vi "motion_generate_test_withvelocitycontrol_withswingdelay.vi"() -> ()   [LabVIEW 2017]
uses:
  d2619827-b21f-489f-b2a3-d550c82ff8e2.vi
  Downloads/Interfacing File 1/Software_Driver/DynamixelSDK/DynamixelSDK-master/labview/dxl_x86_c.lvlib/dxl_x86_c.lvlib
panel:
  in  "millisecond timer value":u32=200
  in  "ADDR_MX_GOAL_Velocity 2":u8=5
  in  "data 4":u16
  in  "data 3":u16
  in  "data 2":u16
  in  "data":u16
  in  "ADDR_MX_GOAL_Velocity":u8=5
  in  "angle 2":dbl=180.0
  in  "swing 2":dbl=185.0
  in  "motor3 2":dbl=220.0
  in  "motor1&2 2":dbl=150.0
  in  "z축 선택":dbl
  in  "motor1&2":dbl=150.0
  in  "motor3":dbl=220.0
  in  "swing":dbl=185.0
  in  "angle":dbl=180.0
  in  "Boolean":bool
  in  "positioning time_2":u32
  in  "positioning time_1":u32
  in  "initial_5":dbl=230.0
  in  "initial_4":dbl=180.0
  out "value : MX (knob)\npresent position 5":u16(knob)
  out "value : MX (knob)\npresent position 4":u16(knob)
  in  "dynamixel_id 5":u8=5
  in  "dynamixel_id 4":u8=4
  out "protocol_version 2":dbl=2.0
  in  "ADDR_MX_\nPRESENT_POSITION 2":u16=132
  out "dynamixel_error 2":string
  out "dynamixel_comm_result  2":string
  in  "ADDR_MX_\nGOAL_POSITION 2":u16=116
  in  "ADDR_MX_\nTORQUE_ENABLE 2":u16=64
  in  "initial_3":dbl=260.0
  in  "initial_1&2":dbl=230.0
  out "value : MX (knob)\npresent position 3":u16(knob)
  out "value : MX (knob)\npresent position 2":u16(knob)
  out "value : MX (knob)\npresent position":u16(knob)
  in  "dynamixel_id 3":u8=3
  in  "dynamixel_id 2":u8=2
  out "dynamixel_comm_result":string
  out "dynamixel_error":string
  in  "device_name":string="COM3"
  in  "ADDR_MX_\nPRESENT_POSITION":u16=36
  in  "ADDR_MX_\nGOAL_POSITION":u16=30
  in  "ADDR_MX_\nTORQUE_ENABLE":u16=24
  out "protocol_version":dbl=1.0
  in  "terminate":bool
  out "port_num":i32
  in  "dynamixel_id":u8=1
  in  "baud_rate":i32=57600
  # "Motor connection status"
  # "Time set"
  # "Sensing data"
  # "Handler setup"
  # "link length"
  # "initial angle"
  # "desired angle"
  # "*각 관절에 모터 연결 시 180도 라인 기준으로 연결 시키기 \n(-각도 반영해주기 위함!) \n-> 모터 input은 -180~180까지 계산됨!"
  # "*yaw motor는 0도 라인 기준으로 연결 시키기"
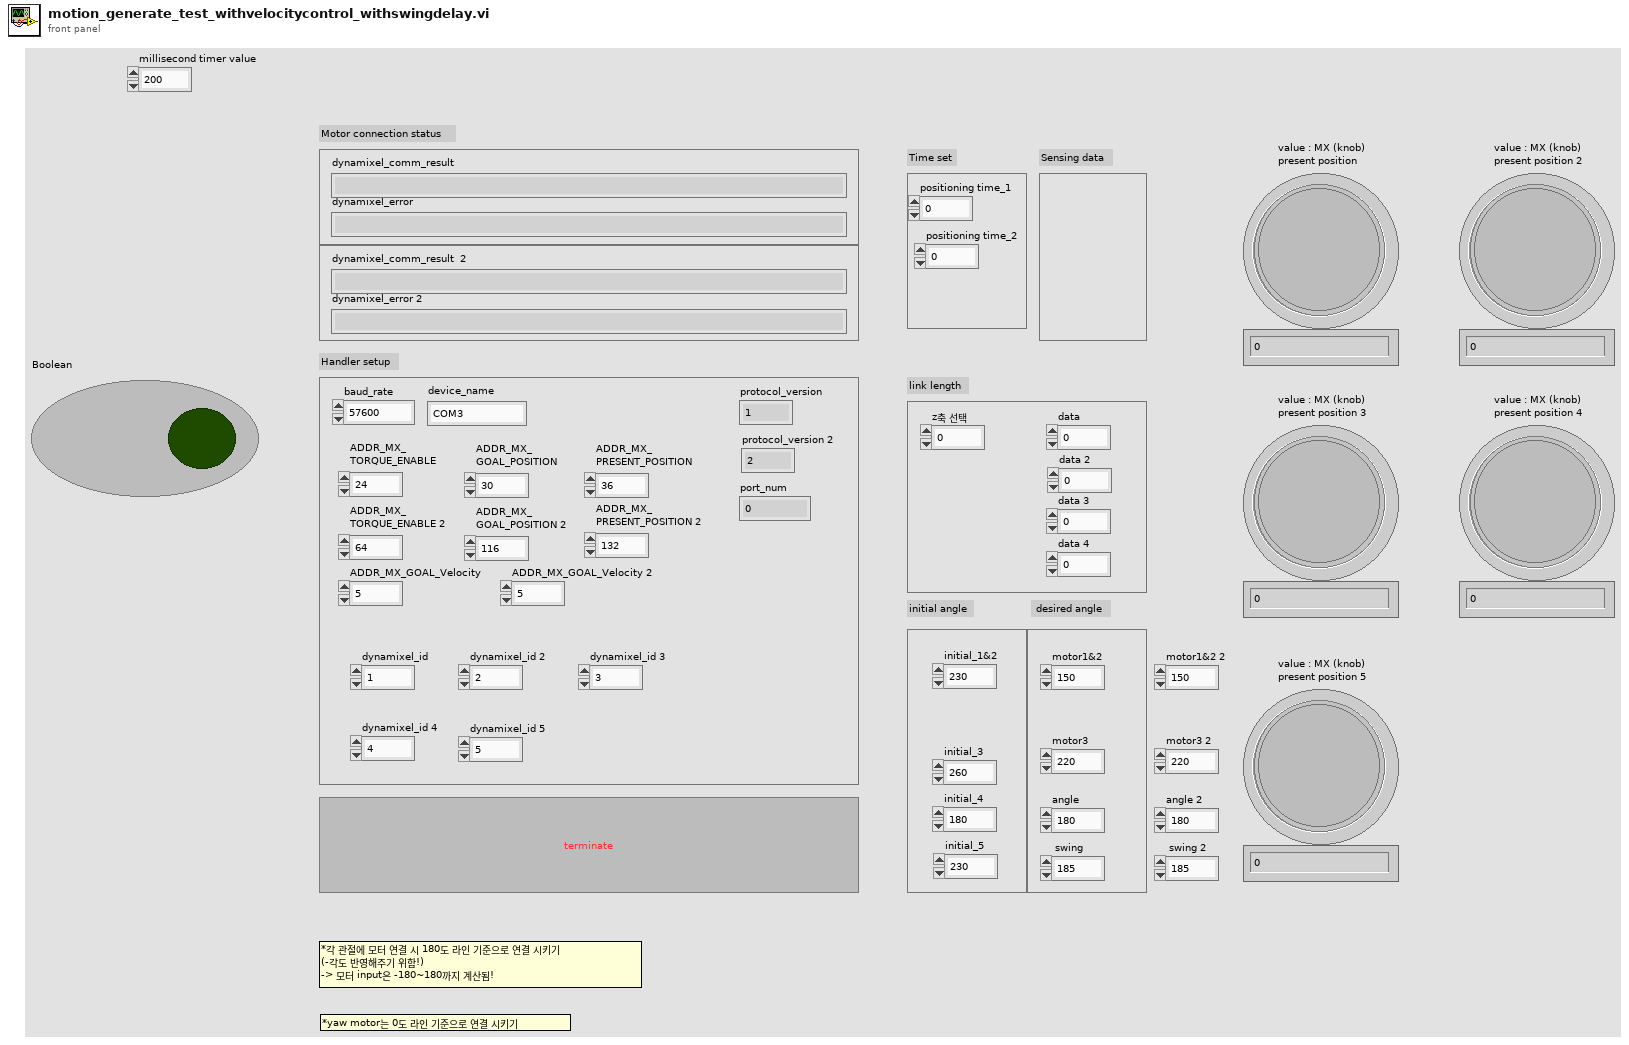
[diagram p1: front panel]
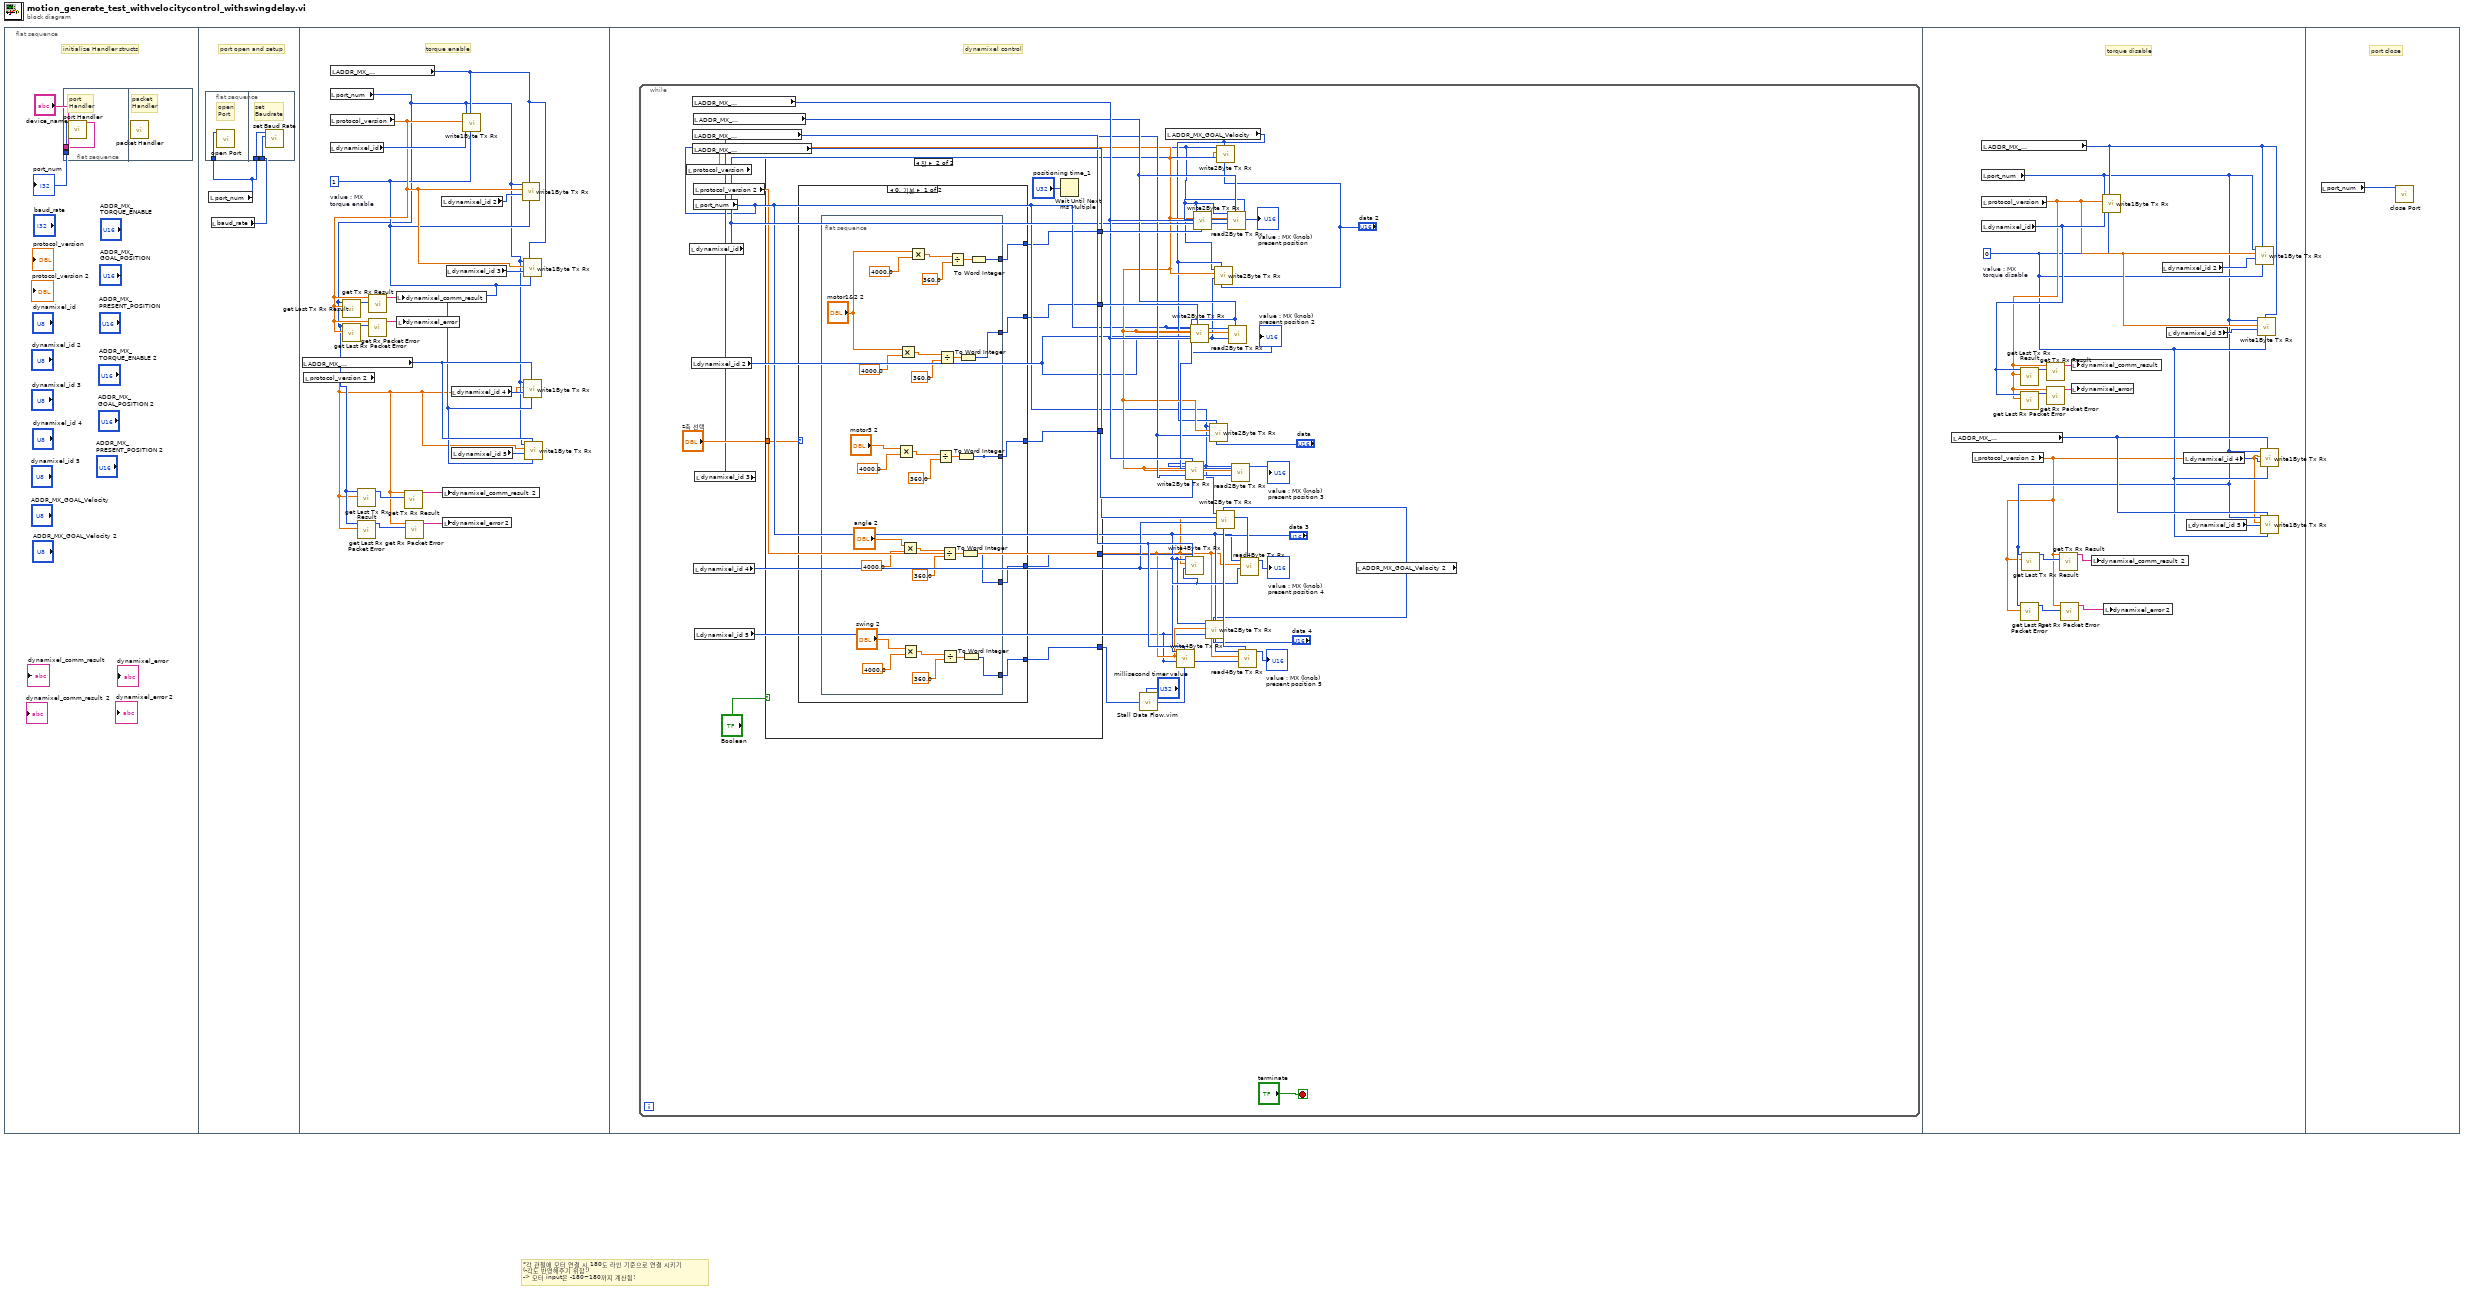
[diagram p0: block diagram]
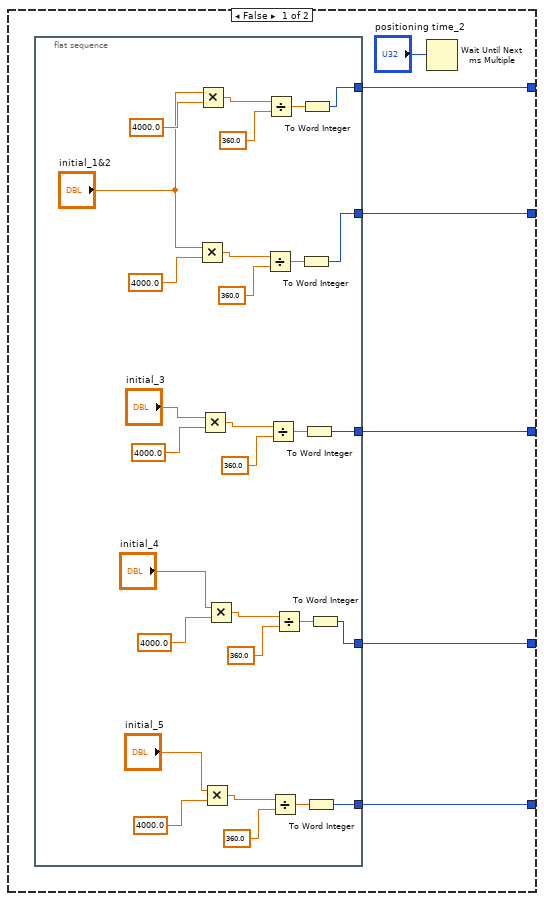
[diagram p2: hidden frame]
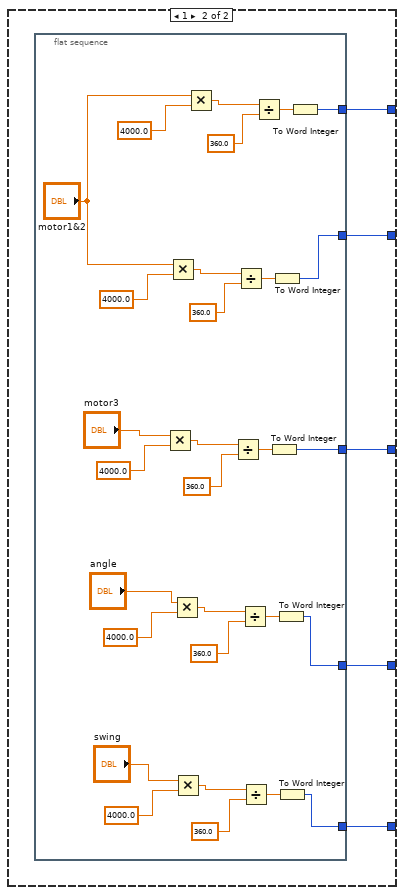
[diagram p3: hidden frame]
diagram:
  # "*각 관절에 모터 연결 시 180도 라인 기준으로 연결 시키기 \n(-각도 반영해주기 위함!) \n-> 모터 input은 -180~180까지 계산됨!"
  n1 = flat-sequence {
    frame #0 {
      # "initialize Handler structs"
      n2 = flat-sequence {
        tunnel: [w4] -> w2
        tunnel: "device_name" -> [w3]
        frame #0 {
          # "port\nHandler"
          n3 = call "port Handler.vi"("port_name"=w3) -> ("function return"=w4:i32)  [unwired: 10 in]
        }
        frame #1 {
          # "packet\nHandler"
          n4 = call "packet Handler.vi"() -> ()  [unwired: 12 in]
        }
      }
      "port_num" <- w2
    }
    frame #1 {
      # "port open and setup"
      n5 = flat-sequence {
        tunnel: w6 -> [w7]
        tunnel: w6 -> [w9]
        tunnel: w5 -> [w8]
        frame #0 {
          # "open\nPort"
          n6 = call "open Port.vi"("port_num"=w7) -> ()  [unwired: 10 in, 1 out]
        }
        frame #1 {
          # "set\nBaudrate"
          n7 = call "set Baud Rate.vi"("baudrate"=w8, "port_num"=w9) -> ()  [unwired: 9 in, 1 out]
        }
      }
      n8 = local read "port_num"() -> (w6:i32)
      n9 = local read "baud_rate"() -> (w5:i32)
    }
    frame #2 {
      w16 = 1  # value : MX torque enable
      # "torque enable"
      n10 = local read "ADDR_MX_\nTORQUE_ENABLE 2"() -> (w17:u16)
      n11 = local read "protocol_version 2"() -> (w10:dbl)
      n12 = local read "port_num"() -> (w11:i32)
      n13 = local read "protocol_version"() -> (w21:dbl)
      n14 = local read "dynamixel_id"() -> (w28:u8)
      n15 = local read "ADDR_MX_\nTORQUE_ENABLE"() -> (w20:u16)
      n16 = call "get Last Tx Rx Result.vi"("protocol_version"=w21, "port_num"=w11) -> ("function return"=w24:i32)  [unwired: 9 in]
      n17 = call "get Last Rx Packet Error.vi"("protocol_version"=w21, "port_num"=w11) -> ("function return"=w25:u8)  [unwired: 9 in]
      n18 = call "get Last Rx Packet Error.vi"("protocol_version"=w10, "port_num"=w11) -> ("function return"=w13:u8)  [unwired: 9 in]
      n19 = call "get Last Tx Rx Result.vi"("protocol_version"=w10, "port_num"=w11) -> ("function return"=w15:i32)  [unwired: 9 in]
      n20 = call "get Rx Packet Error.vi"("error"=w25, "protocol_version"=w21) -> ("function return"=w27:string)  [unwired: 9 in]
      n21 = call "get Tx Rx Result.vi"("result"=w24, "protocol_version"=w21) -> ("function return"=w26:string)  [unwired: 9 in]
      n22 = local write "dynamixel_comm_result"(w26) -> ()
      n23 = local write "dynamixel_error"(w27) -> ()
      n24 = call "get Tx Rx Result.vi"("result"=w15, "protocol_version"=w10) -> ("function return"=w14:string)  [unwired: 9 in]
      n25 = call "get Rx Packet Error.vi"("error"=w13, "protocol_version"=w10) -> ("function return"=w12:string)  [unwired: 9 in]
      n26 = local read "dynamixel_id 2"() -> (w23:u8)
      n27 = local write "dynamixel_comm_result  2"(w14) -> ()
      n28 = local write "dynamixel_error 2"(w12) -> ()
      n29 = local read "dynamixel_id 3"() -> (w22:u8)
      n30 = local read "dynamixel_id 4"() -> (w19:u8)
      n31 = local read "dynamixel_id 5"() -> (w18:u8)
      n32 = call "write1Byte Tx Rx.vi"("data"=w16, "address"=w20, "id"=w28, "protocol_version"=w21, "port_num"=w11) -> ()  [unwired: 7 in]
      n33 = call "write1Byte Tx Rx.vi"("data"=w16, "address"=w20, "id"=w23, "protocol_version"=w21, "port_num"=w11) -> ()  [unwired: 7 in]
      n34 = call "write1Byte Tx Rx.vi"("data"=w16, "address"=w20, "id"=w22, "protocol_version"=w21, "port_num"=w11) -> ()  [unwired: 7 in]
      n35 = call "write1Byte Tx Rx.vi"("data"=w16, "address"=w17, "id"=w19, "protocol_version"=w10, "port_num"=w11) -> ()  [unwired: 7 in]
      n36 = call "write1Byte Tx Rx.vi"("data"=w16, "address"=w17, "id"=w18, "protocol_version"=w10, "port_num"=w11) -> ()  [unwired: 7 in]
    }
    frame #3 {
      # "dynamixel control"
      n37 = while {
        stop <- "terminate" stop-if-true
        n38 = local read "protocol_version"() -> (w42:dbl)
        n39 = local read "dynamixel_id"() -> (w43:u8)
        n40 = local read "dynamixel_id 2"() -> (w41:u8)
        n41 = local read "ADDR_MX_\nGOAL_POSITION"() -> (w58:u16)
        n42 = local read "ADDR_MX_\nGOAL_POSITION 2"() -> (w49:u16)
        n43 = local read "ADDR_MX_\nPRESENT_POSITION 2"() -> (w50:u16)
        n44 = local read "ADDR_MX_\nPRESENT_POSITION"() -> (w57:u16)
        n45 = local read "protocol_version 2"() -> (w34:dbl)
        n46 = local read "port_num"() -> (w35:i32)
        n47 = local read "dynamixel_id 4"() -> (w39:u8)
        n48 = local read "dynamixel_id 5"() -> (w33:u8)
        n49 = local read "dynamixel_id 3"() -> (w45:u8)
        n50 = case shown="참" "Boolean" {
          tunnel: [w67 w103] -> w60
          tunnel: [w66 w102] -> w59
          tunnel: [w65 w101] -> w56
          tunnel: [w64 w99] -> w48
          tunnel: [w63 w100] -> w31
          tunnel: "z축 선택" -> [_ w97]
          frame False {
            n51 = flat-sequence {
              tunnel: [w92] -> w67
              tunnel: [w82] -> w66
              tunnel: [w81] -> w65
              tunnel: [w72] -> w64
              tunnel: [w71] -> w63
              frame #0 {
                n52 = Multiply(x="initial_1&2", y=4000.0) -> (x*y=w90:dbl)
                n53 = Multiply(x="initial_1&2", y=4000.0) -> (x*y=w95:dbl)
                n54 = Multiply(x="initial_3", y=4000.0) -> (x*y=w86:dbl)
                n55 = Multiply(x="initial_5", y=4000.0) -> (x*y=w75:dbl)
                n56 = Multiply(x="initial_4", y=4000.0) -> (x*y=w79:dbl)
                n57 = Divide(x=w90, y=360.0) -> (x/y=w88:dbl)
                n58 = Divide(x=w95, y=360.0) -> (x/y=w93:dbl)
                n59 = Divide(x=w86, y=360.0) -> (x/y=w84:dbl)
                n60 = Divide(x=w75, y=360.0) -> (x/y=w73:dbl)
                n61 = Divide(x=w79, y=360.0) -> (x/y=w77:dbl)
                n62 = To Word Integer(number=w88) -> (16bit integer=w82:i16)
                n63 = To Word Integer(number=w93) -> (16bit integer=w92:i16)
                n64 = To Word Integer(number=w84) -> (16bit integer=w81:i16)
                n65 = To Word Integer(number=w73) -> (16bit integer=w71:i16)
                n66 = To Word Integer(number=w77) -> (16bit integer=w72:i16)
              }
            }
            n67 = Wait Until Next ms Multiple(millisecond multiple="positioning time_2") -> ()  [unwired: 1 out]
          }
          frame True {
            n68 = case shown="0, 기본" w97 {
              tunnel: [w104 w142] -> w103
              tunnel: [w105 w141] -> w102
              tunnel: [w106 w140] -> w101
              tunnel: [w107 w139] -> w100
              tunnel: [w108 w138] -> w99
              frame 0, Default {
                n69 = flat-sequence {
                  tunnel: [w133] -> w104
                  tunnel: [w128] -> w105
                  tunnel: [w109] -> _
                  tunnel: [w115] -> w107
                  tunnel: [w114] -> w108
                  tunnel: [w109] -> w106
                  frame #0 {
                    n70 = Multiply(x="motor3 2", y=4000.0) -> (x*y=w126:dbl)
                    n71 = Multiply(x="motor1&2 2", y=4000.0) -> (x*y=w131:dbl)
                    n72 = Multiply(x="angle 2", y=4000.0) -> (x*y=w122:dbl)
                    n73 = Multiply(x="swing 2", y=4000.0) -> (x*y=w118:dbl)
                    n74 = Multiply(x="motor1&2 2", y=4000.0) -> (x*y=w136:dbl)
                    n75 = Divide(x=w126, y=360.0) -> (x/y=w124:dbl)
                    n76 = Divide(x=w131, y=360.0) -> (x/y=w129:dbl)
                    n77 = Divide(x=w122, y=360.0) -> (x/y=w120:dbl)
                    n78 = Divide(x=w118, y=360.0) -> (x/y=w116:dbl)
                    n79 = Divide(x=w136, y=360.0) -> (x/y=w134:dbl)
                    n80 = To Word Integer(number=w124) -> (16bit integer=w109:i16)
                    n81 = To Word Integer(number=w129) -> (16bit integer=w128:i16)
                    n82 = To Word Integer(number=w120) -> (16bit integer=w114:i16)
                    n83 = To Word Integer(number=w116) -> (16bit integer=w115:i16)
                    n84 = To Word Integer(number=w134) -> (16bit integer=w133:i16)
                  }
                }
              }
              frame 1 {
                n85 = flat-sequence {
                  tunnel: [w167] -> w142
                  tunnel: [w162] -> w141
                  tunnel: [w157] -> w140
                  tunnel: [w148] -> w139
                  tunnel: [w147] -> w138
                  frame #0 {
                    n86 = Multiply(x="motor3", y=4000.0) -> (x*y=w160:dbl)
                    n87 = Multiply(x="motor1&2", y=4000.0) -> (x*y=w165:dbl)
                    n88 = Multiply(x="angle", y=4000.0) -> (x*y=w155:dbl)
                    n89 = Multiply(x="swing", y=4000.0) -> (x*y=w151:dbl)
                    n90 = Multiply(x="motor1&2", y=4000.0) -> (x*y=w170:dbl)
                    n91 = Divide(x=w160, y=360.0) -> (x/y=w158:dbl)
                    n92 = Divide(x=w165, y=360.0) -> (x/y=w163:dbl)
                    n93 = Divide(x=w155, y=360.0) -> (x/y=w153:dbl)
                    n94 = Divide(x=w151, y=360.0) -> (x/y=w149:dbl)
                    n95 = Divide(x=w170, y=360.0) -> (x/y=w168:dbl)
                    n96 = To Word Integer(number=w158) -> (16bit integer=w157:i16)
                    n97 = To Word Integer(number=w163) -> (16bit integer=w162:i16)
                    n98 = To Word Integer(number=w153) -> (16bit integer=w147:i16)
                    n99 = To Word Integer(number=w149) -> (16bit integer=w148:i16)
                    n100 = To Word Integer(number=w168) -> (16bit integer=w167:i16)
                  }
                }
              }
            }
            n101 = Wait Until Next ms Multiple(millisecond multiple="positioning time_1") -> ()  [unwired: 1 out]
          }
        }
        n102 = call "Stall Data Flow.vim"("value in"=w31, "milliseconds to wait"="millisecond timer value") -> ("value out"=w30:i16)  [unwired: 1 out]
        n103 = local read "ADDR_MX_GOAL_Velocity"() -> (w36:u8)
        n104 = call "write4Byte Tx Rx.vi"("data"=w30, "address"=w49, "id"=w33, "protocol_version"=w34, "port_num"=w35) -> ()  [unwired: 7 in]
        n105 = call "write2Byte Tx Rx.vi"("data"=w56, "address"=w58, "id"=w45, "protocol_version"=w42, "port_num"=w35) -> ()  [unwired: 7 in]
        n106 = call "write4Byte Tx Rx.vi"("data"=w48, "address"=w49, "id"=w39, "protocol_version"=w34, "port_num"=w35) -> ()  [unwired: 7 in]
        n107 = call "write2Byte Tx Rx.vi"("data"=w59, "address"=w58, "id"=w41, "protocol_version"=w42, "port_num"=w35) -> ()  [unwired: 7 in]
        n108 = call "write2Byte Tx Rx.vi"("data"=w60, "address"=w58, "id"=w43, "protocol_version"=w42, "port_num"=w35) -> ()  [unwired: 7 in]
        n109 = call "write2Byte Tx Rx.vi"("data"="data", "address"=w36, "id"=w45, "protocol_version"=w42, "port_num"=w35) -> ()  [unwired: 7 in]
        n110 = call "write2Byte Tx Rx.vi"("data"="data 2", "address"=w36, "id"=w41, "protocol_version"=w42, "port_num"=w35) -> ()  [unwired: 7 in]
        n111 = call "write2Byte Tx Rx.vi"("data"="data 2", "address"=w36, "id"=w43, "protocol_version"=w42, "port_num"=w35) -> ()  [unwired: 7 in]
        n112 = call "read2Byte Tx Rx.vi"("address"=w57, "id"=w43, "protocol_version"=w42, "port_num"=w35) -> ("function return"=→"value : MX (knob)\npresent position":u16)  [unwired: 7 in]
        n113 = call "read2Byte Tx Rx.vi"("address"=w57, "id"=w41, "protocol_version"=w42, "port_num"=w35) -> ("function return"=→"value : MX (knob)\npresent position 2":u16)  [unwired: 7 in]
        n114 = call "read2Byte Tx Rx.vi"("address"=w57, "id"=w45, "protocol_version"=w42, "port_num"=w35) -> ("function return"=→"value : MX (knob)\npresent position 3":u16)  [unwired: 7 in]
        n115 = call "read4Byte Tx Rx.vi"("address"=w50, "id"=w33, "protocol_version"=w34, "port_num"=w35) -> ("function return"=→"value : MX (knob)\npresent position 5":u32)  [unwired: 7 in]
        n116 = call "read4Byte Tx Rx.vi"("address"=w50, "id"=w39, "protocol_version"=w34, "port_num"=w35) -> ("function return"=→"value : MX (knob)\npresent position 4":u32)  [unwired: 7 in]
        n117 = local read "ADDR_MX_GOAL_Velocity 2"() -> (w32:u8)
        n118 = call "write2Byte Tx Rx.vi"("data"="data 4", "address"=w32, "id"=w33, "protocol_version"=w34, "port_num"=w35) -> ()  [unwired: 7 in]
        n119 = call "write2Byte Tx Rx.vi"("data"="data 3", "address"=w32, "id"=w39, "protocol_version"=w34, "port_num"=w35) -> ()  [unwired: 7 in]
      }
    }
    frame #4 {
      w178 = 0  # value : MX torque disable
      # "torque disable"
      n120 = local read "ADDR_MX_\nTORQUE_ENABLE 2"() -> (w179:u16)
      n121 = local read "protocol_version 2"() -> (w174:dbl)
      n122 = local read "port_num"() -> (w176:i32)
      n123 = local read "ADDR_MX_\nTORQUE_ENABLE"() -> (w182:u16)
      n124 = local read "protocol_version"() -> (w183:dbl)
      n125 = local read "dynamixel_id"() -> (w186:u8)
      n126 = call "get Last Rx Packet Error.vi"("protocol_version"=w174, "port_num"=w176) -> ("function return"=w175:u8)  [unwired: 9 in]
      n127 = call "get Last Tx Rx Result.vi"("protocol_version"=w183, "port_num"=w186) -> ("function return"=w188:i32)  [unwired: 9 in]
      n128 = call "get Last Rx Packet Error.vi"("protocol_version"=w183, "port_num"=w186) -> ("function return"=w187:u8)  [unwired: 9 in]
      n129 = call "get Last Tx Rx Result.vi"("protocol_version"=w174, "port_num"=w176) -> ("function return"=w177:i32)  [unwired: 9 in]
      n130 = call "get Tx Rx Result.vi"("result"=w188, "protocol_version"=w183) -> ("function return"=w189:string)  [unwired: 9 in]
      n131 = call "get Rx Packet Error.vi"("error"=w187, "protocol_version"=w183) -> ("function return"=w190:string)  [unwired: 9 in]
      n132 = call "get Tx Rx Result.vi"("result"=w177, "protocol_version"=w174) -> ("function return"=w172:string)  [unwired: 9 in]
      n133 = call "get Rx Packet Error.vi"("error"=w175, "protocol_version"=w174) -> ("function return"=w173:string)  [unwired: 9 in]
      n134 = local write "dynamixel_comm_result"(w189) -> ()
      n135 = local write "dynamixel_error"(w190) -> ()
      n136 = local write "dynamixel_comm_result  2"(w172) -> ()
      n137 = call "write1Byte Tx Rx.vi"("data"=w178, "address"=w182, "id"=w186, "protocol_version"=w183, "port_num"=w176) -> ()  [unwired: 7 in]
      n138 = local write "dynamixel_error 2"(w173) -> ()
      n139 = local read "dynamixel_id 2"() -> (w185:u8)
      n140 = local read "dynamixel_id 3"() -> (w184:u8)
      n141 = local read "dynamixel_id 4"() -> (w180:u8)
      n142 = local read "dynamixel_id 5"() -> (w181:u8)
      n143 = call "write1Byte Tx Rx.vi"("data"=w178, "address"=w182, "id"=w185, "protocol_version"=w183, "port_num"=w176) -> ()  [unwired: 7 in]
      n144 = call "write1Byte Tx Rx.vi"("data"=w178, "address"=w182, "id"=w184, "protocol_version"=w183, "port_num"=w176) -> ()  [unwired: 7 in]
      n145 = call "write1Byte Tx Rx.vi"("data"=w178, "address"=w179, "id"=w180, "protocol_version"=w174, "port_num"=w176) -> ()  [unwired: 7 in]
      n146 = call "write1Byte Tx Rx.vi"("data"=w178, "address"=w179, "id"=w181, "protocol_version"=w174, "port_num"=w176) -> ()  [unwired: 7 in]
    }
    frame #5 {
      # "port close"
      n147 = local read "port_num"() -> (w191:i32)
      n148 = call "close Port.vi"("port_num"=w191) -> ()  [unwired: 11 in]
    }
  }
